vi "_errorHandler.vi"(8 "error in (no error)":errorcluster, 10 "Additional Text":string, 11 "Error Type":T1) -> (0 "error out":errorcluster)   [LabVIEW 2013, in "BSON.lvlib"]
uses:
  BSON.lvlib
  status.ctl
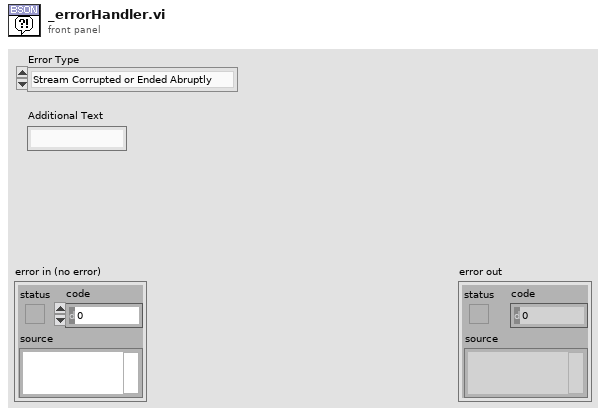
[diagram p1: front panel]
types:
  T1 = typedef "BSON.lvlib/status.ctl" = enum16{"Stream Corrupted or Ended Abruptly", "Incorrect Type In Stream", "ObjectID Invalid", "Method Not Implemented", "Invalid Name", "Invalid URI", "AutoReconnect", "Operation Failed", "Incorrectly Configured", "Cursor Not Found", "Timeout", "Invalid Type", "Empty Name", "Duplicate Name", "MD5Incorrect"}
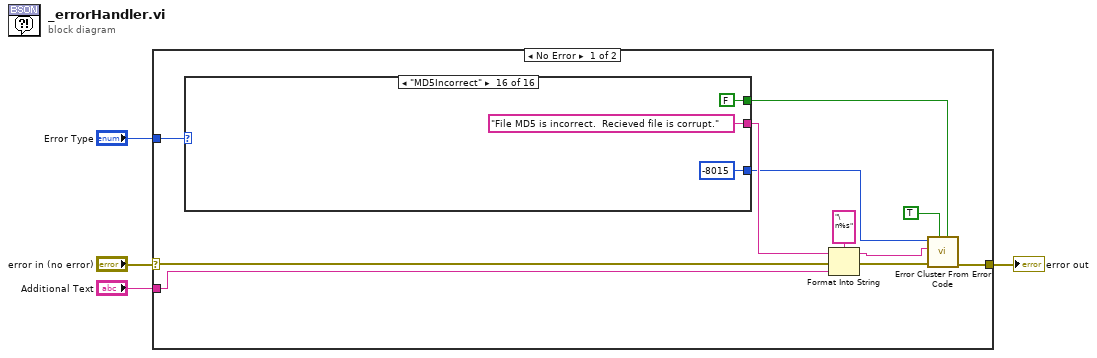
[diagram p0: block diagram]
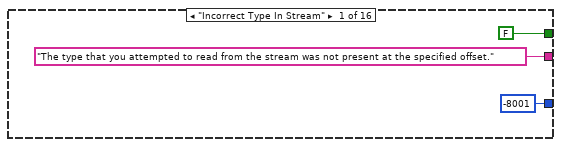
[diagram p2: hidden frame]
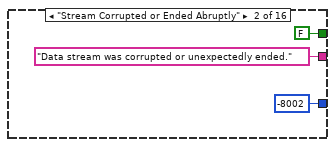
[diagram p3: hidden frame]
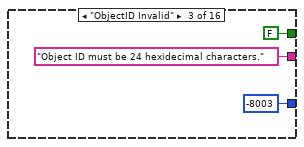
[diagram p4: hidden frame]
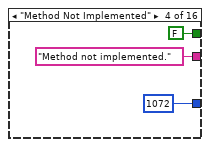
[diagram p5: hidden frame]
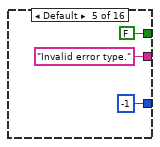
[diagram p6: hidden frame]
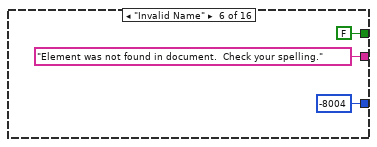
[diagram p7: hidden frame]
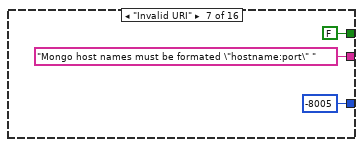
[diagram p8: hidden frame]
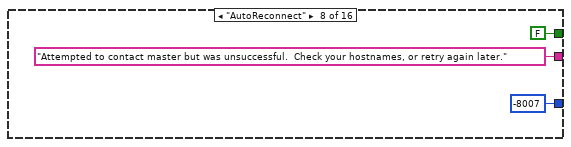
[diagram p9: hidden frame]
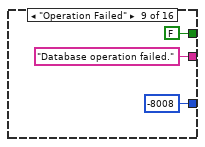
[diagram p10: hidden frame]
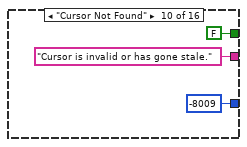
[diagram p11: hidden frame]
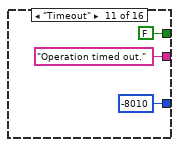
[diagram p12: hidden frame]
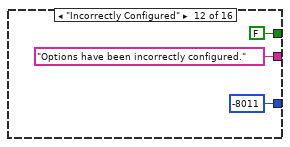
[diagram p13: hidden frame]
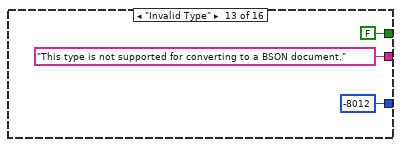
[diagram p14: hidden frame]
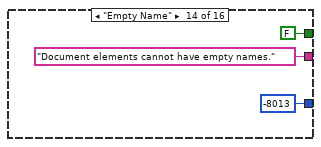
[diagram p15: hidden frame]
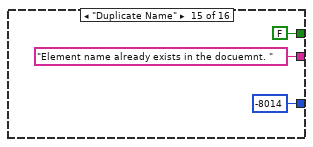
[diagram p16: hidden frame]
diagram:
  n1 = case shown="No Error" "error in (no error)" {
    selector: "error in (no error)" -> [w11 w64]
    tunnel: [w14 w64] -> w3
    tunnel: "Error Type" -> [w15 _]
    tunnel: "Additional Text" -> [w6 _]
    frame No Error {
      n2 = case shown="\"MD5Incorrect\"" w15 {
        tunnel: ["The type that you attempted to read from the stream was not present at the specified offset." "Data stream was corrupted or unexpectedly ended." "Object ID must be 24 hexidecimal characters." "Method not implemented." "Invalid error type." "Element was not found in document.  Check your spelling." "Mongo host names must be formated \"hostname:port\" " "Attempted to contact master but was unsuccessful.  Check your hostnames, or retry again later." "Database operation failed." "Cursor is invalid or has gone stale." "Operation timed out." "Options have been incorrectly configured." "This type is not supported for converting to a BSON document." "Document elements cannot have empty names." "Element name already exists in the docuemnt. " "File MD5 is incorrect.  Recieved file is corrupt."] -> w8
        tunnel: [FALSE FALSE FALSE FALSE FALSE FALSE FALSE FALSE FALSE FALSE FALSE FALSE FALSE FALSE FALSE FALSE] -> w12
        tunnel: [-8001 ("error code (0)") -8002 ("error code (0)") -8003 ("error code (0)") 1072 ("error code (0)") -1 ("error code (0)") -8004 ("error code (0)") -8005 ("error code (0)") -8007 ("error code (0)") -8008 ("error code (0)") -8009 ("error code (0)") -8010 ("error code (0)") -8011 ("error code (0)") -8012 ("error code (0)") -8013 ("error code (0)") -8014 ("error code (0)") -8015 ("error code (0)")] -> w5
        frame "Incorrect Type In Stream" {
        }
        frame "Stream Corrupted or Ended Abruptly" {
        }
        frame "ObjectID Invalid" {
        }
        frame "Method Not Implemented" {
        }
        frame Default {
        }
        frame "Invalid Name" {
        }
        frame "Invalid URI" {
        }
        frame "AutoReconnect" {
        }
        frame "Operation Failed" {
        }
        frame "Cursor Not Found" {
        }
        frame "Timeout" {
        }
        frame "Incorrectly Configured" {
        }
        frame "Invalid Type" {
        }
        frame "Empty Name" {
        }
        frame "Duplicate Name" {
        }
        frame "MD5Incorrect" {
        }
      }
      n3 = Format Into String(format string="\n%s", initial string=w8, error in=w11, w6) -> (resulting string=w7:string, error out=w10:errorcluster)
      n4 = call <vilib>:"Error Cluster From Error Code.vi"("is warning? (False)"=w12, "show call chain? (False)"=TRUE, "error in (no error)"=w10, "error message (\"\")"=w7, "error code (0)"=w5) -> ("error out"=w14:errorcluster)  [unwired: 4 in]
    }
    frame Error {
    }
  }
  "error out" <- w3
